vi "Global 1.vi"() -> ()   [LabVIEW 2015]
panel:
  in  "charged":bool
  in  "i":bool
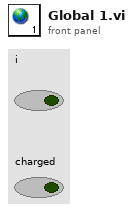
[diagram p1: front panel]
diagram:
